vi "Configure Multi Eval Meas List Segment Tx Power.vi"(6 "Enable (Off)":bool, 7 "Statistics (20)":i32=20, 8 "error in (no error)":errorcluster, 9 "Segment (1)":i32=1, 10 "Instance (1)":T1=1, 11 "VISA resource name":refnum<visa-resource-name>) -> (0 "error out":errorcluster, 3 "VISA resource name out":refnum<visa-resource-name>)   [LabVIEW 2020, in "Rohde&Schwarz CMWXP NR FR1 Measurement.lvlib"]
doc: "Defines settings for the measurement of the total TX power for segment <no>.\n\nAttribute:\nRSCMWXPNRFR1M_ATTR_MULTI_EVAL_MEAS_LIST_SEGMENT_TX_POWER\n\nRemote-control command:\nCONFigure:NRSub:MEAS<i>:MEValuation:LIST:SEGMent<no>:POWer"
uses:
  <instrlib>/Rohde&Schwarz CMWXP NR FR1 Measurement/Rohde&Schwarz CMWXP NR FR1 Measurement.lvlib
  <instrlib>/Rohde&Schwarz CMWXP NR FR1 Measurement/Private/_Instance.ctl
  <instrlib>/Rohde&Schwarz CMWXP NR FR1 Measurement/Private/rsidr_core.llb/rsidr_core.lvlib
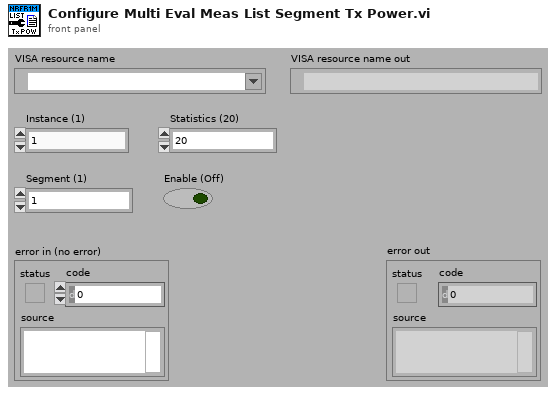
[diagram p1: front panel]
types:
  T1 = typedef "Rohde&Schwarz CMWXP NR FR1 Measurement.lvlib/_Instance.ctl" = i32
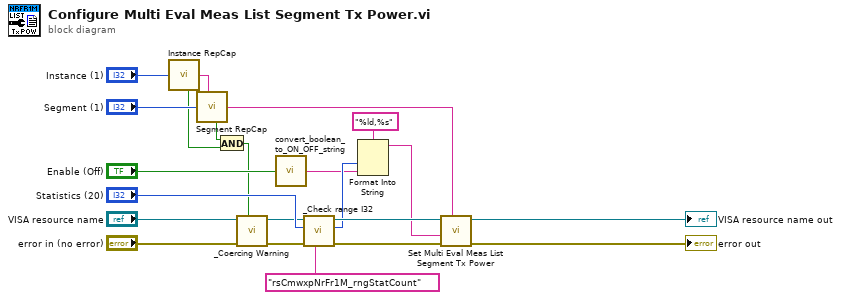
[diagram p0: block diagram]
diagram:
  n1 = call <instrlib>:"Instance RepCap.vi"("Instance In"="Instance (1)") -> ("In Range?"=w2:bool, "RepCap Identifier Out"=w20:string)  [unwired: 1 in]
  n2 = call <instrlib>:"Segment RepCap.vi"("Segment In"="Segment (1)", "RepCap String In (\"\")"=w20) -> ("In Range?"=w1:bool, "RepCap Identifier Out"=w17:string)
  n3 = And(x=w1, y=w2) -> (x .and. y?=w3:bool)
  n4 = call <instrlib>:"_Coercing Warning.vi"("In Range?"=w3, "error in (no error)"="error in (no error)", "VISA resource name"="VISA resource name") -> ("error out"=w5:errorcluster, "VISA resource name out"=w4:refnum<visa-resource-name>)  [unwired: 7 in]
  n5 = call <instrlib>:"convert_boolean_to_ON_OFF_string.vi"("boolean value in"="Enable (Off)") -> ("string value out"=w9:string)  [unwired: 4 in]
  n6 = call <instrlib>:"_Check range I32.vi"("Range Table Identifier"="rsCmwxpNrFr1M_rngStatCount", "error in (no error)"=w5, "I32 Value In"="Statistics (20)", "VISA resource name"=w4) -> ("error out"=w12:errorcluster, "I32 Value Out"=w10:i32, "VISA resource name out"=w13:refnum<visa-resource-name>)  [unwired: 5 in]
  n7 = Format Into String(format string="%ld,%s", w10, w9) -> (resulting string=w8:string)  [unwired: 2 in, 1 out]
  n8 = call "Set Multi Eval Meas List Segment Tx Power"("Repeated Capabilities"=w17, "error in (no error)"=w12, "Multi Eval Meas List Segment Tx Power ()"=w8, "instrument handle"=w13) -> ("error out"=→"error out":errorcluster, "instrument handle out"=→"VISA resource name out":refnum<visa-resource-name>)  [unwired: 6 in]
